vi "test Get-Set-Get Parameter Definitions.vi"(8 "error in":errorcluster, 11 "TestCase in":refnum<class "Scripting.lvclass">) -> (0 "error out":errorcluster, 3 "TestCase out":refnum<class "Scripting.lvclass">)   [LabVIEW 2020, in "Scripting.lvclass"]
uses:
  Scripting.lvclass
  C:/dev/git/niveristand-custom-device-testing-tools/VeriStandScriptingTestCase/VeriStandScriptingTestCase.lvclass
  Shared/1553 Channel.ctl
  Shared/Address.ctl
  Shared/Major Frame Definition.ctl
  Shared/Minor Frame Definition.ctl
  Shared/Message Definition.ctl
  Shared/Message Type.ctl
  Shared/Terminal Endpoint.ctl
  Shared/Parameter Definition.ctl
  niveristand-custom-device-testing-tools/VeriStandScriptingTestCase/VeriStandScriptingTestCase.lvclass/VeriStandScriptingTestCase.ctl
  niveristand-custom-device-testing-tools/VeriStandScriptingTestCase/Read Target.vi
  NationalInstruments.VeriStand.SystemDefinitionAPI
  <vilib>/addons/_JKI Toolkits/VI Tester/TestCase.llb/TestCase.lvclass
  Scripting/AIM MIL-STD-1553 Scripting.lvlib
  C:/Program Files (x86)/National Instruments/LabVIEW 2020/vi.lib/addons/_JKI Toolkits/VI Tester/TestCase.llb/TestCase.lvclass
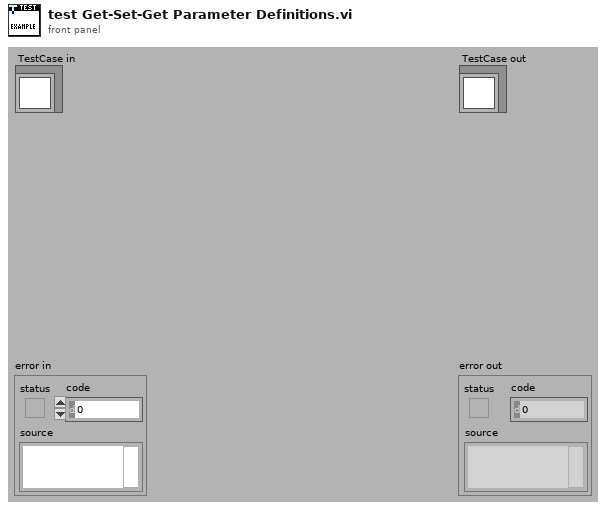
[diagram p1: front panel]
types:
  T1 = typedef "1553 Channel.ctl" = cluster{"HW channel":u16, "terminal addresses":T2[], "terminal names":string[], "acyclic frame names":string[], "major frames":T3[], "minor frames":T4[], "messages":T5[]}
  T2 = typedef "Address.ctl" = u16
  T3 = typedef "Major Frame Definition.ctl" = cluster{"name":string, "minor frames":string[]}
  T4 = typedef "Minor Frame Definition.ctl" = cluster{"name":string, "messages":string[]}
  T5 = typedef "Message Definition.ctl" = cluster{"name":string, "message type":T6, "endpoint Tx":T7, "endpoint Rx":T7, "create timestamp channel":bool, "mode code":u16, "number of words":u16, "parameters":cluster{"name":string, "default value":dbl, "unit":string, "parameter definition":T8}[]}
  T6 = typedef "Message Type.ctl" = string
  T7 = typedef "Terminal Endpoint.ctl" = cluster{"terminal address":T2, "subaddress":T2}
  T8 = typedef "Parameter Definition.ctl" = cluster{"start index":i32, "size (bits)":i32, "encoding":enum16{"BNR", "BCD", "Discrete"}, "signed":bool, "multiplier":dbl, "offset":dbl}
  T9 = typedef "Custom Device API.lvlib/Custom Device Item Ref.ctl" = u64
  T10 = cluster{"name":string, "default value":dbl, "unit":string, "parameter definition":T8}[]
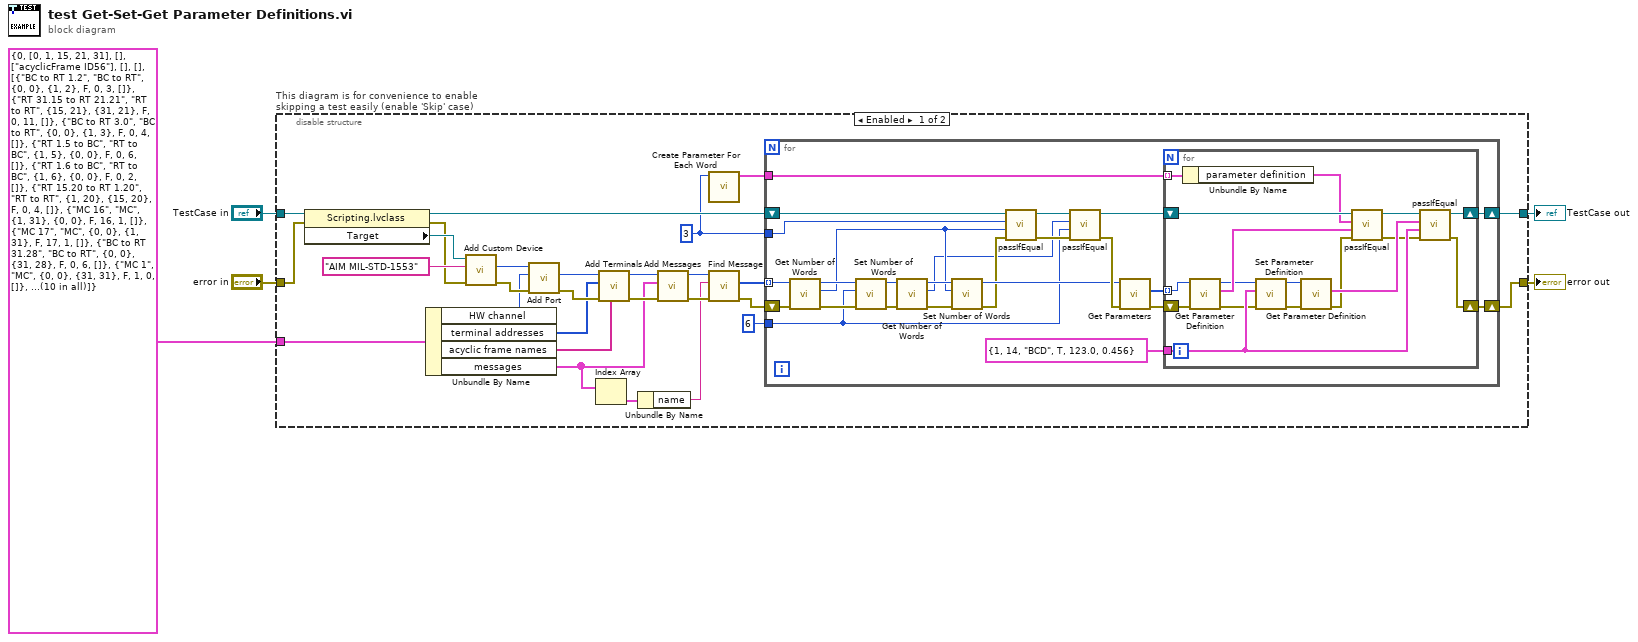
[diagram p0: block diagram]
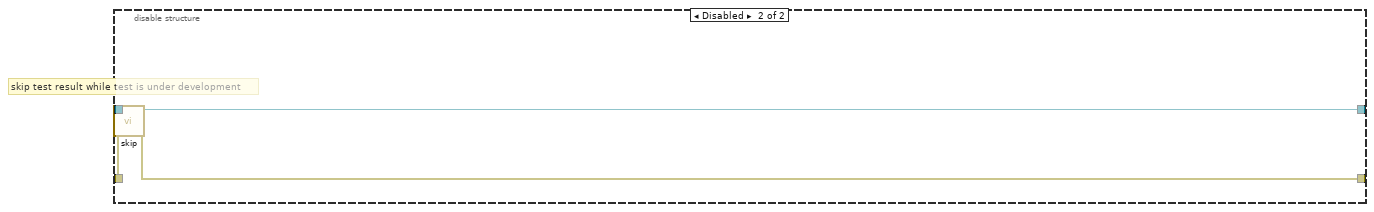
[diagram p2: hidden frame]
diagram:
  n1 = disable-structure "This diagram is for convenience to enable skipping a test easily (enable 'Skip' case)" shown="Enabled" {
    disable-tunnel: "TestCase in" -> [w32 w79]
    disable-tunnel: [w10 w77] -> w2
    disable-tunnel: [w9 w78] -> w4
    disable-tunnel: "error in" -> [w14 w76]
    disable-tunnel: T1 {"HW channel"=0, "terminal addresses"=[0, 1, 15, 21, 31], "terminal names"=[], "acyclic frame names"=["acyclicFrame ID56"], "major frames"=[], "minor frames"=[], "messages"=[{"name"="BC to RT 1.2", "message type"="BC to RT", "endpoint Tx"={"terminal address"=0, "subaddress"=0}, "endpoint Rx"={"terminal address"=1, "subaddress"=2}, "create timestamp channel"=FALSE, "mode code"=0, "number of words"=3, "parameters"=[]}, {"name"="RT 31.15 to RT 21.21", "message type"="RT to RT", "endpoint Tx"={"terminal address"=15, "subaddress"=21}, "endpoint Rx"={"terminal address"=31, "subaddress"=21}, "create timestamp channel"=FALSE, "mode code"=0, "number of words"=11, "parameters"=[]}, {"name"="BC to RT 3.0", "message type"="BC to RT", "endpoint Tx"={"terminal address"=0, "subaddress"=0}, "endpoint Rx"={"terminal address"=1, "subaddress"=3}, "create timestamp channel"=FALSE, "mode code"=0, "number of words"=4, "parameters"=[]}, {"name"="RT 1.5 to BC", "message type"="RT to BC", "endpoint Tx"={"terminal address"=1, "subaddress"=5}, "endpoint Rx"={"terminal address"=0, "subaddress"=0}, "create timestamp channel"=FALSE, "mode code"=0, "number of words"=6, "parameters"=[]}, {"name"="RT 1.6 to BC", "message type"="RT to BC", "endpoint Tx"={"terminal address"=1, "subaddress"=6}, "endpoint Rx"={"terminal address"=0, "subaddress"=0}, "create timestamp channel"=FALSE, "mode code"=0, "number of words"=2, "parameters"=[]}, {"name"="RT 15.20 to RT 1.20", "message type"="RT to RT", "endpoint Tx"={"terminal address"=1, "subaddress"=20}, "endpoint Rx"={"terminal address"=15, "subaddress"=20}, "create timestamp channel"=FALSE, "mode code"=0, "number of words"=4, "parameters"=[]}, {"name"="MC 16", "message type"="MC", "endpoint Tx"={"terminal address"=1, "subaddress"=31}, "endpoint Rx"={"terminal address"=0, "subaddress"=0}, "create timestamp channel"=FALSE, "mode code"=16, "number of words"=1, "parameters"=[]}, {"name"="MC 17", "message type"="MC", "endpoint Tx"={"terminal address"=0, "subaddress"=0}, "endpoint Rx"={"terminal address"=1, "subaddress"=31}, "create timestamp channel"=FALSE, "mode code"=17, "number of words"=1, "parameters"=[]}, {"name"="BC to RT 31.28", "message type"="BC to RT", "endpoint Tx"={"terminal address"=0, "subaddress"=0}, "endpoint Rx"={"terminal address"=31, "subaddress"=28}, "create timestamp channel"=FALSE, "mode code"=0, "number of words"=6, "parameters"=[]}, {"name"="MC 1", "message type"="MC", "endpoint Tx"={"terminal address"=0, "subaddress"=0}, "endpoint Rx"={"terminal address"=31, "subaddress"=31}, "create timestamp channel"=FALSE, "mode code"=1, "number of words"=0, "parameters"=[]}]} ("1553 channel") -> [w6 _]
    frame Enabled {
      w12 = u16 3 ("number of words")
      n2 = property class="Scripting.lvclass"(reference=w32, error in=w14) -> (reference out=w15:refnum<class "Scripting.lvclass">, error out=w13:errorcluster, "Target"=w31:refnum<k24>)
      n3 = Unbundle By Name(w6) -> ("HW channel"=w27:u16, "terminal addresses"=w22:T2[], "acyclic frame names"=w21:string[], "messages"=w7:T5[])
      n4 = call "Add Custom Device.vi"("error in"=w13, "name"="AIM MIL-STD-1553", "target in"=w31) -> ("error out"=w30:errorcluster, "Ballard MIL-STD 1553 custom device"=w29:T9)  [unwired: 6 in, 1 out]
      n5 = call "Add Port.vi"("error in"=w30, "port number"=w27, "custom device ref"=w29) -> ("error out"=w25:errorcluster, "port"=w26:T9)  [unwired: 6 in, 1 out]
      n6 = Index Array(array=w7) -> (element=w18:T5)  [unwired: 1 in]
      n7 = call "Add Terminals.vi"("acyclic frame names"=w21, "error in"=w25, "terminal addresses"=w22, "port in"=w26) -> ("error out"=w23:errorcluster, "port out"=w24:T9)  [unwired: 6 in]
      n8 = Unbundle By Name(w18) -> ("name"=w19:string)
      n9 = call "Add Messages.vi"("error in"=w23, "messages"=w7, "port in"=w24) -> ("error out"=w20:errorcluster, "port out"=w28:T9)  [unwired: 7 in]
      n10 = call "Create Parameter For Each Word.vi"("number of words"=w12) -> ("parameters"=w11:T10)  [unwired: 9 in, 1 out]
      n11 = call "Find Message.vi"("error in"=w20, "message name"=w19, "port in"=w28) -> ("error out"=w16:errorcluster, "message refs"=w17:T9[])  [unwired: 5 in, 2 out]
      n12 = for {
        tunnel: w17 -> [w58] mode=indexing
        shift-right: [w43] -> w9
        shift-left: w16 -> [w57]
        shift-right: [w44] -> w10
        shift-left: w15 -> [w50]
        tunnel: w12 -> [w38]
        tunnel: w11 -> [w46]
        tunnel: u16 6 ("number of words") -> [w35]
        n13 = call "Get Number of Words.vi"("error in"=w57, "message in"=w58) -> ("error out"=w55:errorcluster, "number of words"=w36:u16, "message out"=w56:T9)  [unwired: 7 in]
        n14 = call "Set Number of Words.vi"("error in"=w55, "number of words"=w35, "message in"=w56) -> ("error out"=w54:errorcluster, "message out"=w53:T9)  [unwired: 7 in]
        n15 = call "Get Number of Words.vi"("error in"=w54, "message in"=w53) -> ("error out"=w40:errorcluster, "number of words"=w34:u16, "message out"=w42:T9)  [unwired: 7 in]
        n16 = call "Set Number of Words.vi"("error in"=w40, "number of words"=w36, "message in"=w42) -> ("error out"=w39:errorcluster, "message out"=w41:T9)  [unwired: 7 in]
        n17 = call-dynamic "passIfEqual.vi"("error in (no error)"=w39, "y"=w36, "x"=w38, "TestCase in"=w50) -> ("error out"=w52:errorcluster, "TestCase out"=w51:refnum<class "Scripting.lvclass">)  [unwired: 6 in]
        n18 = call-dynamic "passIfEqual.vi"("error in (no error)"=w52, "y"=w35, "x"=w34, "TestCase in"=w51) -> ("error out"=w49:errorcluster, "TestCase out"=w45:refnum<class "Scripting.lvclass">)  [unwired: 6 in]
        n19 = call "Get Parameters.vi"("error in"=w49, "message in"=w41) -> ("error out"=w48:errorcluster, "parameters"=w47:T9[])  [unwired: 7 in, 1 out]
        n20 = for {
          shift-right: [w64] -> w43
          shift-left: w48 -> [w74]
          tunnel: w47 -> [w75] mode=indexing
          tunnel: w46 -> [w63] mode=indexing
          shift-right: [w65] -> w44
          shift-left: w45 -> [w73]
          tunnel: T8 {"start index"=1, "size (bits)"=14, "encoding"=enum."BCD", "signed"=TRUE, "multiplier"=123.0, "offset"=0.456} ("parameter definition") -> [w67]
          n21 = Unbundle By Name(w63) -> ("parameter definition"=w59:T8)
          n22 = call "Get Parameter Definition.vi"("error in"=w74, "parameter in"=w75) -> ("error out"=w61:errorcluster, "parameter definition"=w72:T8, "parameter out"=w71:T9)  [unwired: 7 in]
          n23 = call "Set Parameter Definition.vi"("error in"=w61, "parameter definition"=w67, "parameter in"=w71) -> ("error out"=w69:errorcluster, "parameter out"=w70:T9)  [unwired: 7 in]
          n24 = call "Get Parameter Definition.vi"("error in"=w69, "parameter in"=w70) -> ("error out"=w60:errorcluster, "parameter definition"=w68:T8)  [unwired: 7 in, 1 out]
          n25 = call-dynamic "passIfEqual.vi"("error in (no error)"=w60, "y"=w72, "x"=w59, "TestCase in"=w73) -> ("error out"=w62:errorcluster, "TestCase out"=w66:refnum<class "Scripting.lvclass">)  [unwired: 6 in]
          n26 = call-dynamic "passIfEqual.vi"("error in (no error)"=w62, "y"=w67, "x"=w68, "TestCase in"=w66) -> ("error out"=w64:errorcluster, "TestCase out"=w65:refnum<class "Scripting.lvclass">)  [unwired: 6 in]
        }
      }
    }
    frame Disabled {
      # "skip test result while test is under development"
      n27 = call <vilib>:"skip.vi"("error in (no error)"=w76, "TestCase in"=w79) -> ("error out"=w78:errorcluster, "TestCase out"=w77:refnum<class "Scripting.lvclass">)  [unwired: 8 in]
    }
  }
  "error out" <- w4
  "TestCase out" <- w2
